vi "Autonomous Independent.vi"() -> ()   [LabVIEW 2016]
doc: "This VI is called when autonomous begins, and will automatically be terminated when autonomous ends. You can carry out timed or sensor driven robot movement independently without needing to return to the caller."
uses:
  <vilib>/Rock Robotics/WPI/Solenoid/WPI_SolenoidValue.ctl
  <vilib>/Rock Robotics/WPI/Utilities/WPI_GetSetVariantRefNum.vi
  <vilib>/Rock Robotics/Network Tables/NT Read String.vi
  <vilib>/Rock Robotics/WPI/RobotDrive/WPI_RobotDriveArcadeDrive_Standard(NoSaturation).vi
  <vilib>/Rock Robotics/Network Tables/NT Write Numeric Array.vi
  <vilib>/Rock Robotics/Network Tables/NT Read Number.vi
  <vilib>/Rock Robotics/WPI/Solenoid/WPI_SolenoidSetEnum.vi
  <vilib>/Rock Robotics/WPI/Solenoid/WPI_SolenoidGetEnum.vi
  <vilib>/addons/control/pid/pid.llb/PID (DBL).vi
  <vilib>/Rock Robotics/Network Tables/NT Write Number.vi
  <vilib>/addons/control/pid/NI_PID_pid.lvlib
panel:
  out "Boolean 3":bool=TRUE
  out "Boolean 2":bool=TRUE
  out "Boolean":bool=TRUE
  # "Be sure to right-click and choose Data Operations>>Make Current Value default if you want to save the array values with the VI"
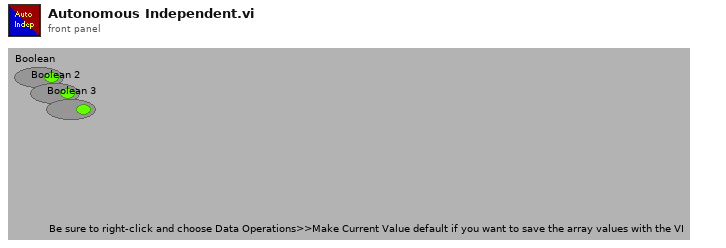
[diagram p1: front panel]
types:
  T1 = typedef "WPI_JoystickDevRef.ctl" = cluster{"Device":T2}
  T2 = typedef "WPI_JoystickDeviceEnum.ctl" = enum16{"USB 0", "USB 1", "USB 2", "USB 3", "USB 4", "USB 5"}
  T3 = typedef "WPI_SolenoidValue.ctl" = enum16{"Off", "On", "Forward", "Reverse"}
  T4 = cluster{"integral time (Ti, min)":dbl, "proportional gain (Kc)":dbl, "derivative time (Td, min)":dbl}
  T5 = cluster{"integral time (Ti, min)":dbl, "proportional gain (Kc)":dbl}
  T6 = typedef "WPI_RobotDriveDevRef.ctl" = cluster{"DevStatus":errorcluster, "Motors[]":T7[], "Square Inputs":bool, "Max Output":dbl}
  T7 = typedef "WPI_MotorControlDeviceRef.ctl" = cluster{"DeviceStatus":errorcluster, "Type":T8, "PWM":cluster{"PWM Channel":T9, "DeadBand":T10}, "CAN":cluster{"Device Number":u8, "SetOutput VI Ref":variant, "GetOutput VI Ref":variant, "Enable VI Ref":variant, "Disable VI Ref":variant, "Data":variant}, "Invert":bool}
  T8 = typedef "WPI_MotorControlType.ctl" = enum16{"PWM", "CAN"}
  T9 = typedef "FPGA_DIOPWMChannel.ctl" = enum8{"PWM 0", "PWM 1", "PWM 2", "PWM 3", "PWM 4", "PWM 5", "PWM 6", "PWM 7", "PWM 8", "PWM 9", "PWM MXP 0", "PWM MXP 1", "PWM MXP 2", "PWM MXP 3", "PWM MXP 4", "PWM MXP 5", "PWM MXP 6", "PWM MXP 7", "PWM MXP 8", "PWM MXP 9", "Invalid"}
  T10 = typedef "WPI_PWMDeadband.ctl" = cluster{"Name":string, "maxPositivePwm":i32, "minPositivePwm":i32, "centerPwm":i32, "maxNegativePwm":i32, "minNegativePwm":i32, "angularRange":u16}
  T11 = typedef "WPI_SolenoidDevRef.ctl" = cluster{"DevStatus":errorcluster, "Pneumatics Control Module":u8, "Forward Solenoid Channel":T12, "Reverse Solenoid Channel":T12}
  T12 = typedef "WPI_SolenoidChannel.ctl" = enum8{"Solenoid 0", "Solenoid 1", "Solenoid 2", "Solenoid 3", "Solenoid 4", "Solenoid 5", "Solenoid 6", "Solenoid 7", "Invalid"}
  T13 = typedef "WPI_GyroDevRef.ctl" = cluster{"DevStatus":errorcluster, "Analog Channel":T14, "Offset":dbl, "Gain (VoltsPerDegree/Second)":dbl, "Gyro Type":enum16{"Analog", "XRS450"}, "Handle":i32, "SPI Bus":T15, "Device Found":bool, "Sample Rate":dbl, "Calibrate On Open":bool}
  T14 = typedef "FPGA_AIChannel.ctl" = enum8{"AI 0", "AI 1", "AI 2", "AI 3", "AI MXP 0", "AI MXP 1", "AI MXP 2", "AI MXP 3", "Invalid"}
  T15 = typedef "spi_bus.ctl" = enum16{"SPI On-Board, CS0", "SPI On-Board, CS1", "SPI On-Board, CS2", "SPI On-Board, CS3", "SPI MXP", "Invalid"}
  T16 = cluster{"Numeric":dbl, "Numeric":dbl, "Numeric":dbl}
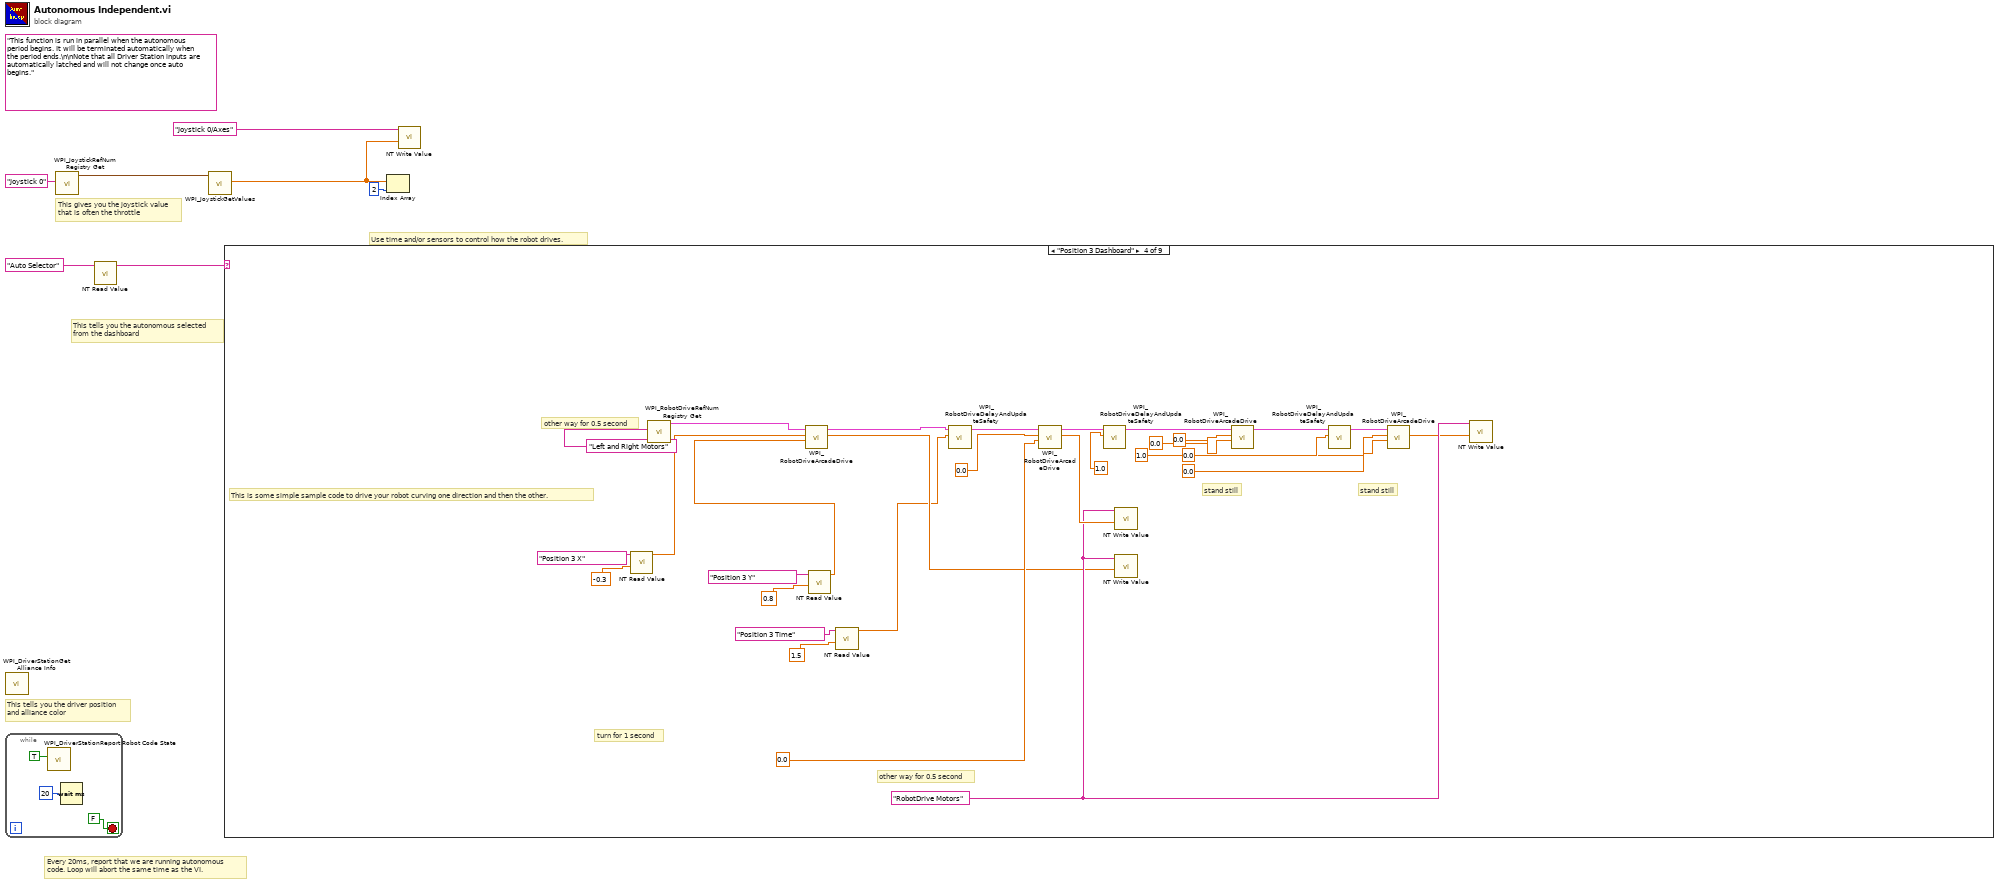
[diagram p0: block diagram]
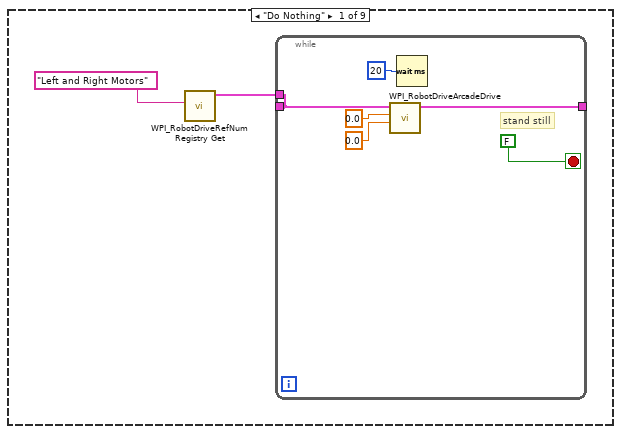
[diagram p2: hidden frame]
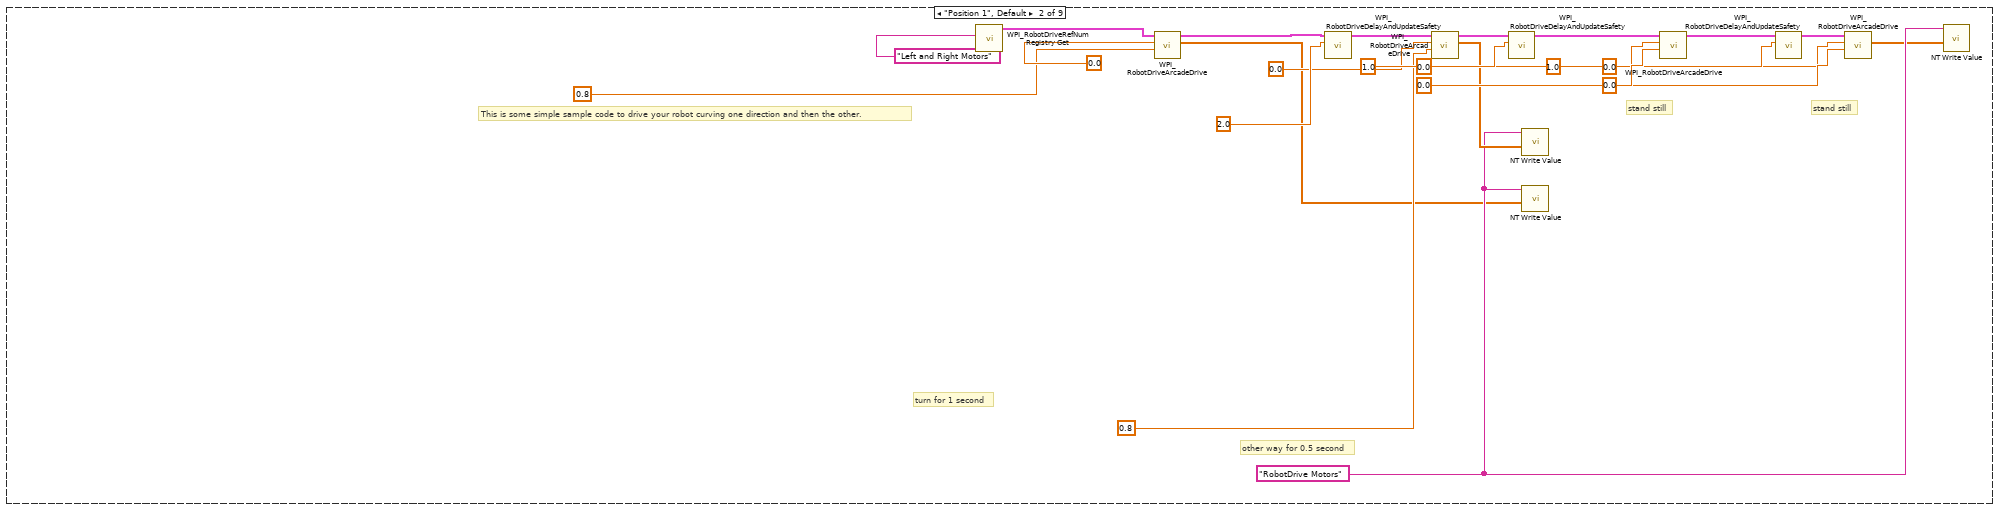
[diagram p3: hidden frame]
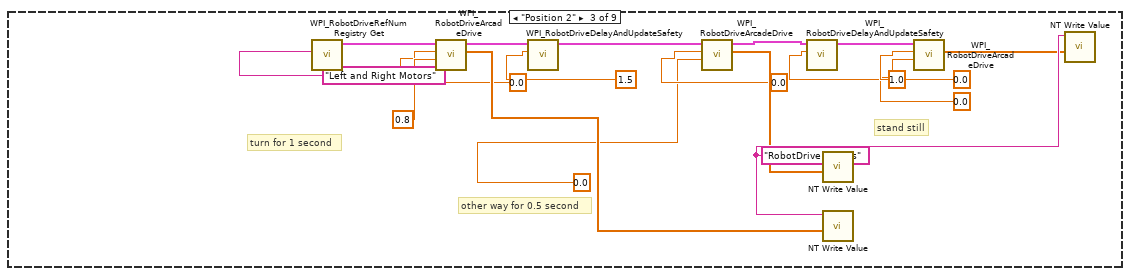
[diagram p4: hidden frame]
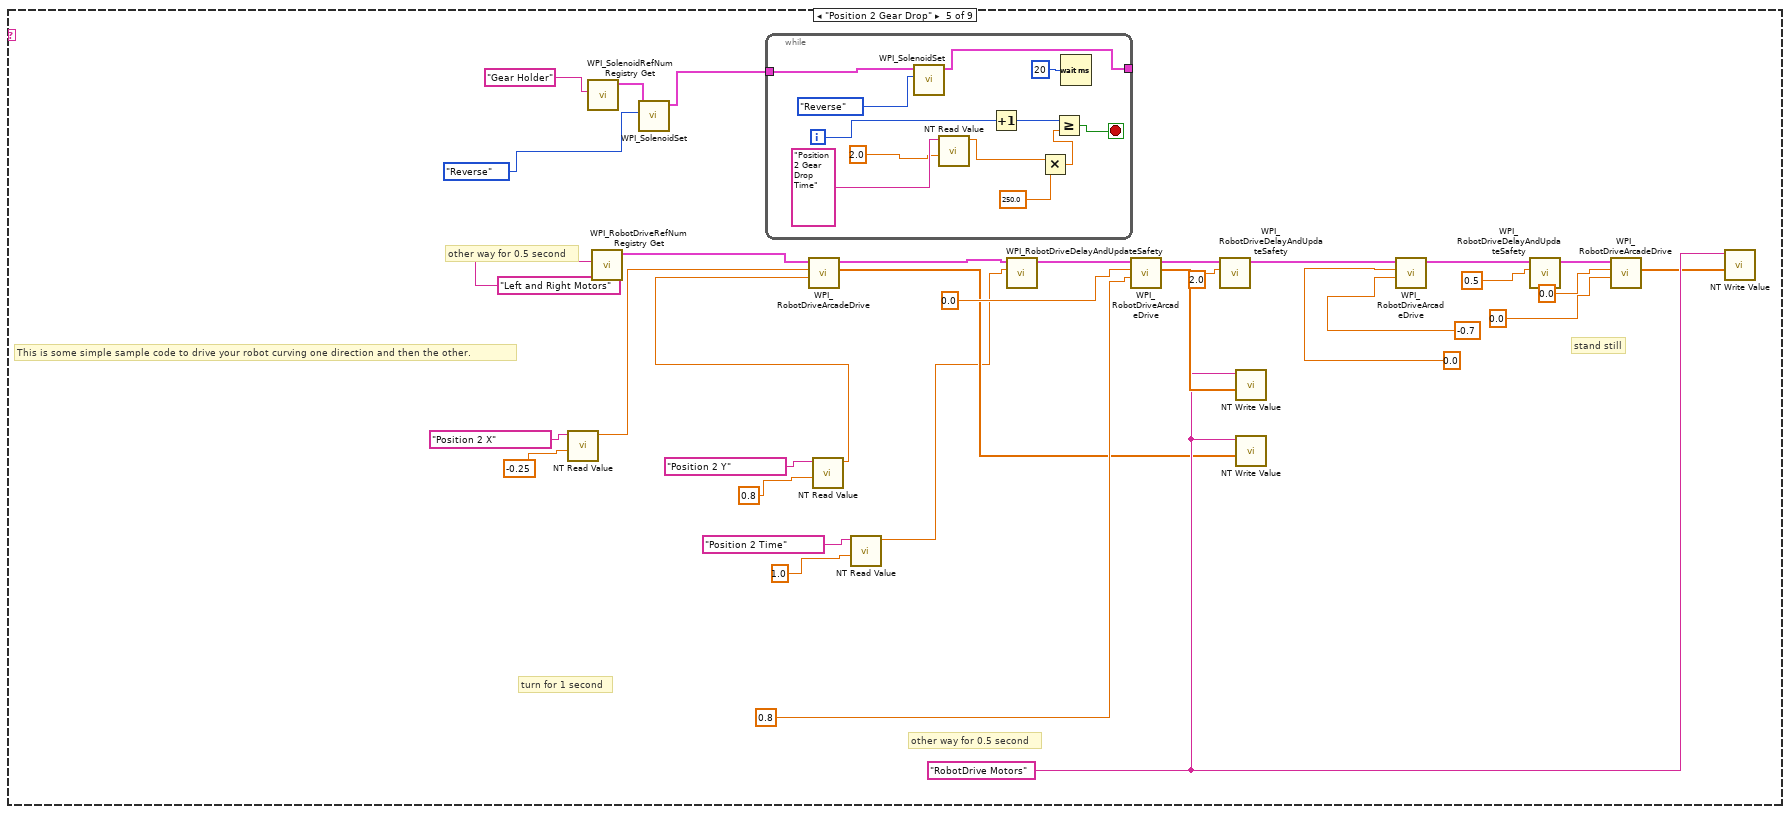
[diagram p5: hidden frame]
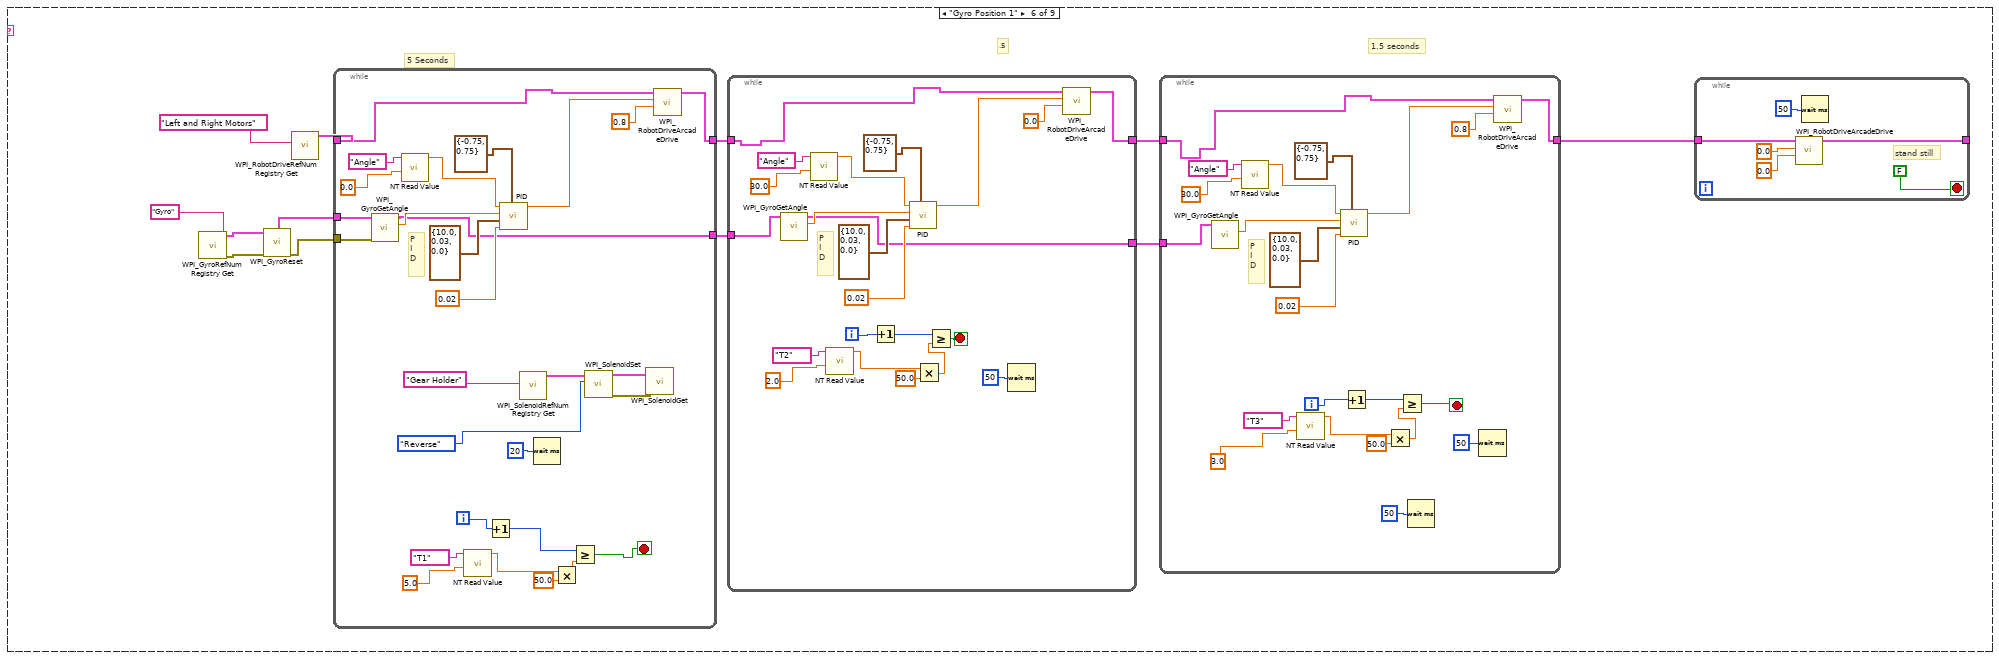
[diagram p6: hidden frame]
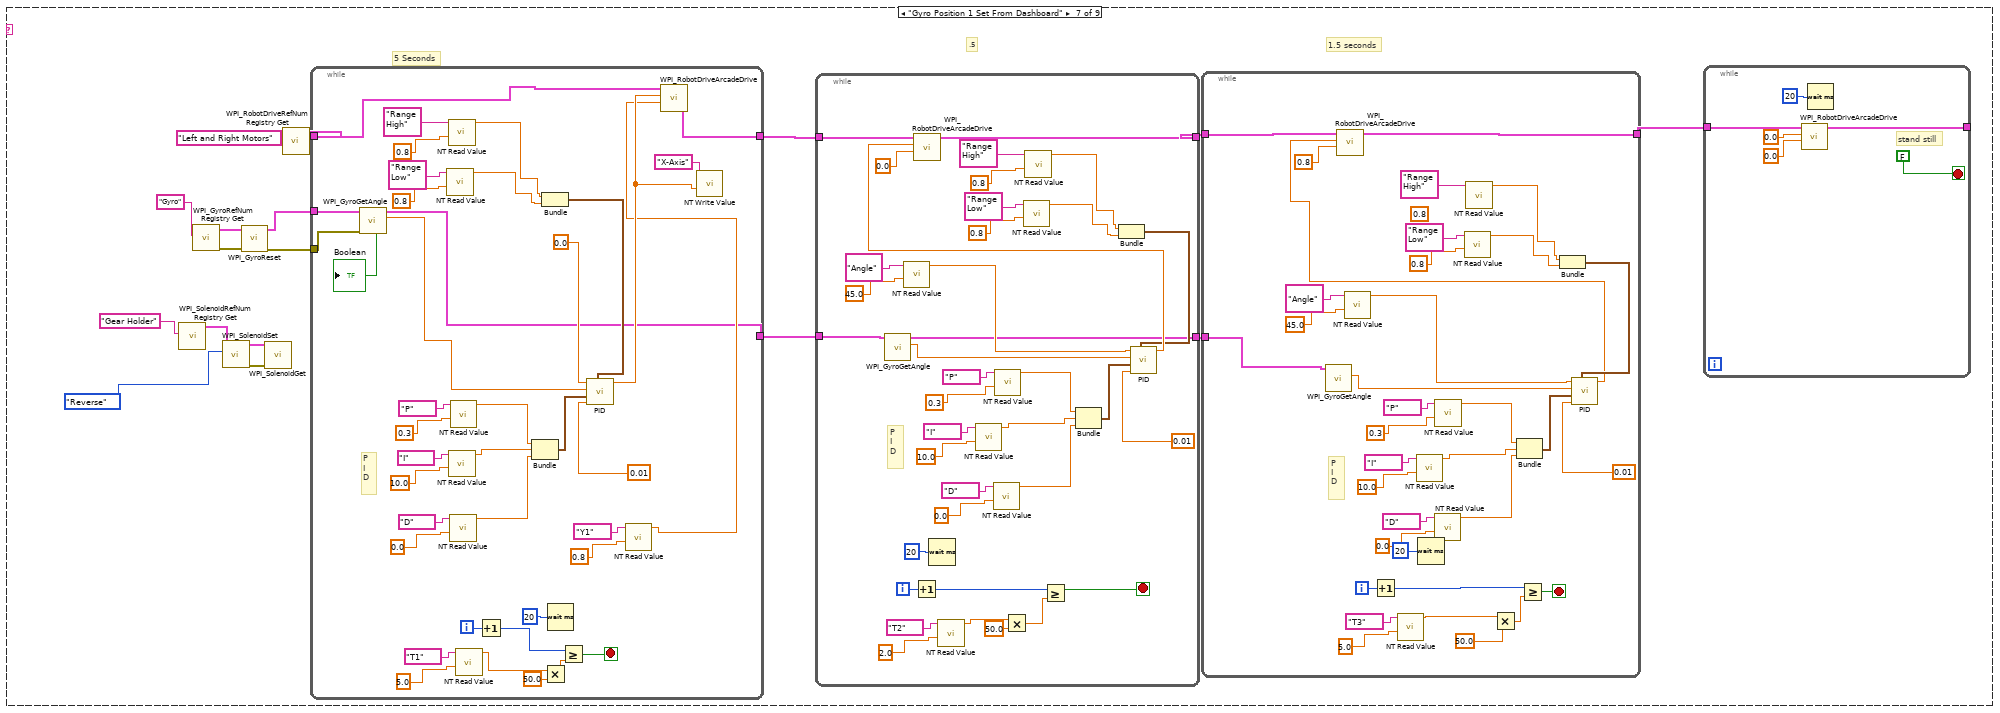
[diagram p7: hidden frame]
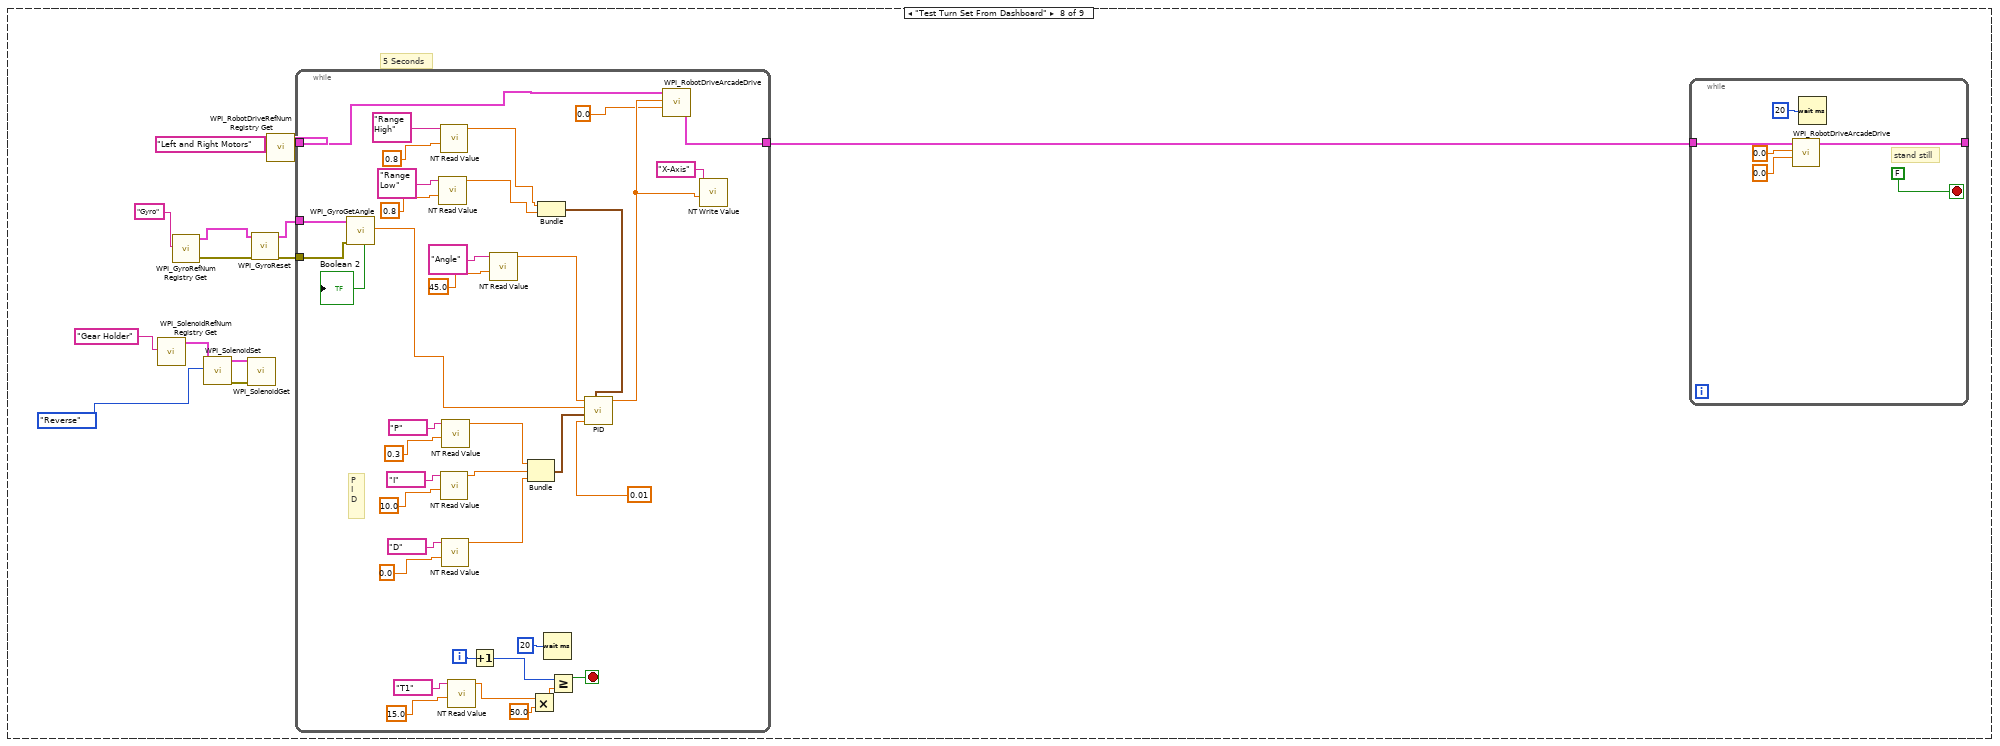
[diagram p8: hidden frame]
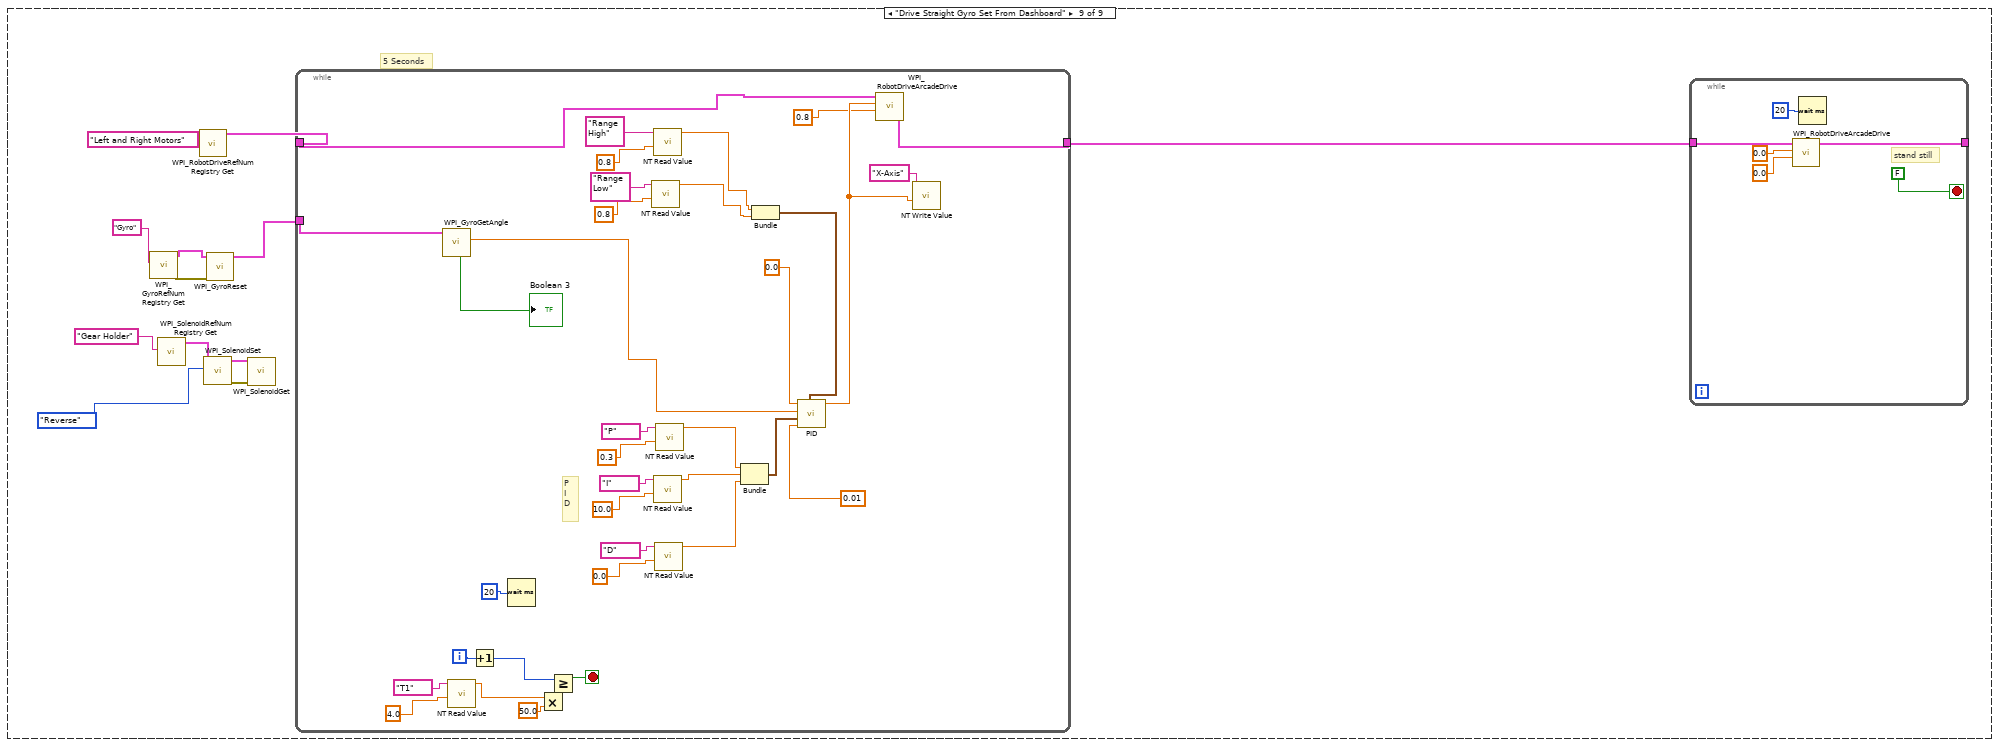
[diagram p9: hidden frame]
diagram:
  (unwired) "This function is run in parallel when the autonomous period begins. It will be terminated automatically when the period ends.\n\nNote that all Driver Station inputs are automatically latched and will not change once auto begins."
  # "This tells you the autonomous selected\nfrom the dashboard"
  # "Every 20ms, report that we are running autonomous\ncode. Loop will abort the same time as the VI."
  # "This gives you the joystick value\nthat is often the throttle"
  # "Use time and/or sensors to control how the robot drives."
  # "This tells you the driver position\nand alliance color"
  n1 = call <vilib>:"WPI_DriverStationGet Alliance Info.vi"() -> ()  [unwired: 12 out]
  n2 = while {
    stop <- FALSE stop-if-true
    n3 = call <vilib>:"WPI_DriverStationReport Robot Code State.vi"("Autonomous"=TRUE) -> ()  [unwired: 10 in, 1 out]
    n4 = Wait (ms)(milliseconds to wait=u32 20) -> ()  [unwired: 1 out]
  }
  n5 = call <vilib>:"WPI_JoystickRefNum Registry Get.vi"("refnum name"="Joystick 0") -> ("JoystickDevRef"=w6:T1)  [unwired: 1 in, 9 out]
  n6 = call-poly <vilib>:"NT Read Value.vi"("Name"="Auto Selector") -> ("String"=w3:string)  [unwired: 9 in, 1 out]
  n7 = call <vilib>:"WPI_JoystickGetValues.vi"("JoystickDevRef"=w6) -> ("Axes"=w2:dbl[])  [unwired: 6 in, 4 out]
  n8 = case shown="\"Position 3 Dashboard\"" w3 {
    frame "Do Nothing" {
      n9 = call <vilib>:"WPI_RobotDriveRefNum Registry Get.vi"("refnum name"="Left and Right Motors") -> ("RobotDriveDevRef"=w11:T6)  [unwired: 1 in, 9 out]
      n10 = while {
        tunnel: [w13] -> _
        tunnel: [w14] -> _
        tunnel: w11 -> [w13]
        stop <- FALSE stop-if-true
        # "stand still"
        n11 = call-poly <vilib>:"WPI_RobotDriveArcadeDrive.vi"("Y axis value"=0.0 ("X axis value"), "X axis value"=0.0, "RobotDriveDevRef"=w13) -> ("RobotDriveDevRef"=w14:T6)  [unwired: 1 in, 7 out]
        n12 = Wait (ms)(milliseconds to wait=20) -> ()  [unwired: 1 out]
      }
    }
    frame "Position 1", Default {
      w26 = "RobotDrive Motors" ("Name")
      # "stand still"
      # "stand still"
      # "other way for 0.5 second"
      # "turn for 1 second"
      # "This is some simple sample code to drive your robot curving one direction and then the other."
      n13 = call <vilib>:"WPI_RobotDriveRefNum Registry Get.vi"("refnum name"="Left and Right Motors") -> ("RobotDriveDevRef"=w41:T6)  [unwired: 1 in, 9 out]
      n14 = call-poly <vilib>:"WPI_RobotDriveArcadeDrive.vi"("Y axis value"=0.8 ("X axis value"), "X axis value"=0.0, "RobotDriveDevRef"=w41) -> ("Motor Values"=w25:dbl[], "RobotDriveDevRef"=w34:T6)  [unwired: 1 in, 6 out]
      n15 = call <vilib>:"WPI_RobotDriveDelayAndUpdateSafety.vi"("Delay (s)"=2.0, "RobotDriveDevRef"=w34) -> ("RobotDriveDevRef 2"=w35:T6)  [unwired: 8 in, 1 out]
      n16 = call-poly <vilib>:"WPI_RobotDriveArcadeDrive.vi"("Y axis value"=0.8 ("X axis value"), "X axis value"=0.0, "RobotDriveDevRef"=w35) -> ("Motor Values"=w27:dbl[], "RobotDriveDevRef"=w36:T6)  [unwired: 1 in, 6 out]
      n17 = call <vilib>:"WPI_RobotDriveDelayAndUpdateSafety.vi"("Delay (s)"=1.0, "RobotDriveDevRef"=w36) -> ("RobotDriveDevRef 2"=w37:T6)  [unwired: 8 in, 1 out]
      n18 = call-poly <vilib>:"NT Write Value.vi"("Numeric Array"=w27, "Name"=w26) -> ()  [unwired: 9 in, 1 out]
      n19 = call-poly <vilib>:"NT Write Value.vi"("Numeric Array"=w25, "Name"=w26) -> ()  [unwired: 9 in, 1 out]
      n20 = call-poly <vilib>:"WPI_RobotDriveArcadeDrive.vi"("Y axis value"=0.0 ("X axis value"), "X axis value"=0.0, "RobotDriveDevRef"=w37) -> ("RobotDriveDevRef"=w23:T6)  [unwired: 1 in, 7 out]
      n21 = call <vilib>:"WPI_RobotDriveDelayAndUpdateSafety.vi"("Delay (s)"=1.0, "RobotDriveDevRef"=w23) -> ("RobotDriveDevRef 2"=w21:T6)  [unwired: 8 in, 1 out]
      n22 = call-poly <vilib>:"WPI_RobotDriveArcadeDrive.vi"("Y axis value"=0.0 ("X axis value"), "X axis value"=0.0, "RobotDriveDevRef"=w21) -> ("Motor Values"=w20:dbl[])  [unwired: 1 in, 7 out]
      n23 = call-poly <vilib>:"NT Write Value.vi"("Numeric Array"=w20, "Name"=w26) -> ()  [unwired: 9 in, 1 out]
    }
    frame "Position 2" {
      w58 = "RobotDrive Motors" ("Name")
      # "stand still"
      # "other way for 0.5 second"
      # "turn for 1 second"
      n24 = call <vilib>:"WPI_RobotDriveRefNum Registry Get.vi"("refnum name"="Left and Right Motors") -> ("RobotDriveDevRef"=w42:T6)  [unwired: 1 in, 9 out]
      n25 = call-poly <vilib>:"WPI_RobotDriveArcadeDrive.vi"("Y axis value"=0.8 ("X axis value"), "X axis value"=0.0, "RobotDriveDevRef"=w42) -> ("Motor Values"=w59:dbl[], "RobotDriveDevRef"=w49:T6)  [unwired: 1 in, 6 out]
      n26 = call <vilib>:"WPI_RobotDriveDelayAndUpdateSafety.vi"("Delay (s)"=1.5, "RobotDriveDevRef"=w49) -> ("RobotDriveDevRef 2"=w48:T6)  [unwired: 8 in, 1 out]
      n27 = call-poly <vilib>:"WPI_RobotDriveArcadeDrive.vi"("Y axis value"=0.0 ("X axis value"), "X axis value"=0.0, "RobotDriveDevRef"=w48) -> ("Motor Values"=w57:dbl[], "RobotDriveDevRef"=w47:T6)  [unwired: 1 in, 6 out]
      n28 = call <vilib>:"WPI_RobotDriveDelayAndUpdateSafety.vi"("Delay (s)"=1.0, "RobotDriveDevRef"=w47) -> ("RobotDriveDevRef 2"=w46:T6)  [unwired: 8 in, 1 out]
      n29 = call-poly <vilib>:"NT Write Value.vi"("Numeric Array"=w57, "Name"=w58) -> ()  [unwired: 9 in, 1 out]
      n30 = call-poly <vilib>:"NT Write Value.vi"("Numeric Array"=w59, "Name"=w58) -> ()  [unwired: 9 in, 1 out]
      n31 = call-poly <vilib>:"WPI_RobotDriveArcadeDrive.vi"("Y axis value"=0.0 ("X axis value"), "X axis value"=0.0, "RobotDriveDevRef"=w46) -> ("Motor Values"=w56:dbl[])  [unwired: 1 in, 7 out]
      n32 = call-poly <vilib>:"NT Write Value.vi"("Numeric Array"=w56, "Name"=w58) -> ()  [unwired: 9 in, 1 out]
    }
    frame "Position 3 Dashboard" {
      w76 = "RobotDrive Motors" ("Name")
      # "stand still"
      # "stand still"
      # "other way for 0.5 second"
      # "turn for 1 second"
      # "This is some simple sample code to drive your robot curving one direction and then the other."
      # "other way for 0.5 second"
      n33 = call-poly <vilib>:"NT Read Value.vi"("Default Value"=-0.3, "Name"="Position 3 X" ("refnum name")) -> ("Numeric"=w66:dbl)  [unwired: 8 in, 1 out]
      n34 = call <vilib>:"WPI_RobotDriveRefNum Registry Get.vi"("refnum name"="Left and Right Motors") -> ("RobotDriveDevRef"=w88:T6)  [unwired: 1 in, 9 out]
      n35 = call-poly <vilib>:"NT Read Value.vi"("Default Value"=0.8, "Name"="Position 3 Y" ("refnum name")) -> ("Numeric"=w63:dbl)  [unwired: 8 in, 1 out]
      n36 = call-poly <vilib>:"WPI_RobotDriveArcadeDrive.vi"("Y axis value"=w63, "X axis value"=w66, "RobotDriveDevRef"=w88) -> ("Motor Values"=w75:dbl[], "RobotDriveDevRef"=w82:T6)  [unwired: 1 in, 6 out]
      n37 = call-poly <vilib>:"NT Read Value.vi"("Default Value"=1.5, "Name"="Position 3 Time" ("refnum name")) -> ("Numeric"=w60:dbl)  [unwired: 8 in, 1 out]
      n38 = call <vilib>:"WPI_RobotDriveDelayAndUpdateSafety.vi"("Delay (s)"=w60, "RobotDriveDevRef"=w82) -> ("RobotDriveDevRef 2"=w83:T6)  [unwired: 8 in, 1 out]
      n39 = call-poly <vilib>:"WPI_RobotDriveArcadeDrive.vi"("Y axis value"=0.0 ("X axis value"), "X axis value"=0.0, "RobotDriveDevRef"=w83) -> ("Motor Values"=w77:dbl[], "RobotDriveDevRef"=w84:T6)  [unwired: 1 in, 6 out]
      n40 = call <vilib>:"WPI_RobotDriveDelayAndUpdateSafety.vi"("Delay (s)"=1.0, "RobotDriveDevRef"=w84) -> ("RobotDriveDevRef 2"=w85:T6)  [unwired: 8 in, 1 out]
      n41 = call-poly <vilib>:"NT Write Value.vi"("Numeric Array"=w77, "Name"=w76) -> ()  [unwired: 9 in, 1 out]
      n42 = call-poly <vilib>:"NT Write Value.vi"("Numeric Array"=w75, "Name"=w76) -> ()  [unwired: 9 in, 1 out]
      n43 = call-poly <vilib>:"WPI_RobotDriveArcadeDrive.vi"("Y axis value"=0.0 ("X axis value"), "X axis value"=0.0, "RobotDriveDevRef"=w85) -> ("RobotDriveDevRef"=w73:T6)  [unwired: 1 in, 7 out]
      n44 = call <vilib>:"WPI_RobotDriveDelayAndUpdateSafety.vi"("Delay (s)"=1.0, "RobotDriveDevRef"=w73) -> ("RobotDriveDevRef 2"=w71:T6)  [unwired: 8 in, 1 out]
      n45 = call-poly <vilib>:"WPI_RobotDriveArcadeDrive.vi"("Y axis value"=0.0 ("X axis value"), "X axis value"=0.0, "RobotDriveDevRef"=w71) -> ("Motor Values"=w70:dbl[])  [unwired: 1 in, 7 out]
      n46 = call-poly <vilib>:"NT Write Value.vi"("Numeric Array"=w70, "Name"=w76) -> ()  [unwired: 9 in, 1 out]
    }
    frame "Position 2 Gear Drop" {
      w109 = "RobotDrive Motors" ("Name")
      # "stand still"
      # "other way for 0.5 second"
      # "turn for 1 second"
      # "This is some simple sample code to drive your robot curving one direction and then the other."
      # "other way for 0.5 second"
      n47 = call-poly <vilib>:"NT Read Value.vi"("Default Value"=-0.25, "Name"="Position 2 X" ("refnum name")) -> ("Numeric"=w99:dbl)  [unwired: 8 in, 1 out]
      n48 = call <vilib>:"WPI_SolenoidRefNum Registry Get.vi"("refnum name"="Gear Holder") -> ("SolenoidDevRef"=w91:T11)  [unwired: 9 in, 1 out]
      n49 = call <vilib>:"WPI_RobotDriveRefNum Registry Get.vi"("refnum name"="Left and Right Motors") -> ("RobotDriveDevRef"=w121:T6)  [unwired: 1 in, 9 out]
      n50 = call-poly <vilib>:"WPI_SolenoidSet.vi"("Value"=WPI_SolenoidValue."Reverse", "SolenoidDevRef"=w91) -> ("SolenoidDevRef"=w89:T11)  [unwired: 8 in, 1 out]
      n51 = while {
        tunnel: w89 -> [w125]
        tunnel: [w123] -> _
        i -> [w127]
        stop <- w122 stop-if-true
        n52 = call-poly <vilib>:"WPI_SolenoidSet.vi"("Value"=WPI_SolenoidValue."Reverse", "SolenoidDevRef"=w125) -> ("SolenoidDevRef"=w123:T11)  [unwired: 8 in, 1 out]
        n53 = call-poly <vilib>:"NT Read Value.vi"("Default Value"=2.0, "Name"="Position 2 Gear Drop Time" ("refnum name")) -> ("Numeric"=w129:dbl)  [unwired: 8 in, 1 out]
        n54 = Increment(x=w127) -> (x+1=w128:i32)
        n55 = Multiply(x=w129, y=250.0) -> (x*y=w133:dbl)
        n56 = Greater Or Equal?(x=w128, y=w133) -> (x >= y?=w122:bool)
        n57 = Wait (ms)(milliseconds to wait=20) -> ()  [unwired: 1 out]
      }
      n58 = call-poly <vilib>:"NT Read Value.vi"("Default Value"=0.8, "Name"="Position 2 Y" ("refnum name")) -> ("Numeric"=w96:dbl)  [unwired: 8 in, 1 out]
      n59 = call-poly <vilib>:"WPI_RobotDriveArcadeDrive.vi"("Y axis value"=w96, "X axis value"=w99, "RobotDriveDevRef"=w121) -> ("Motor Values"=w108:dbl[], "RobotDriveDevRef"=w115:T6)  [unwired: 1 in, 6 out]
      n60 = call-poly <vilib>:"NT Read Value.vi"("Default Value"=1.0, "Name"="Position 2 Time" ("refnum name")) -> ("Numeric"=w93:dbl)  [unwired: 8 in, 1 out]
      n61 = call <vilib>:"WPI_RobotDriveDelayAndUpdateSafety.vi"("Delay (s)"=w93, "RobotDriveDevRef"=w115) -> ("RobotDriveDevRef 2"=w116:T6)  [unwired: 8 in, 1 out]
      n62 = call-poly <vilib>:"WPI_RobotDriveArcadeDrive.vi"("Y axis value"=0.8 ("X axis value"), "X axis value"=0.0, "RobotDriveDevRef"=w116) -> ("Motor Values"=w110:dbl[], "RobotDriveDevRef"=w117:T6)  [unwired: 1 in, 6 out]
      n63 = call <vilib>:"WPI_RobotDriveDelayAndUpdateSafety.vi"("Delay (s)"=2.0, "RobotDriveDevRef"=w117) -> ("RobotDriveDevRef 2"=w118:T6)  [unwired: 8 in, 1 out]
      n64 = call-poly <vilib>:"NT Write Value.vi"("Numeric Array"=w110, "Name"=w109) -> ()  [unwired: 9 in, 1 out]
      n65 = call-poly <vilib>:"NT Write Value.vi"("Numeric Array"=w108, "Name"=w109) -> ()  [unwired: 9 in, 1 out]
      n66 = call-poly <vilib>:"WPI_RobotDriveArcadeDrive.vi"("Y axis value"=-0.7 ("X axis value"), "X axis value"=0.0, "RobotDriveDevRef"=w118) -> ("RobotDriveDevRef"=w106:T6)  [unwired: 1 in, 7 out]
      n67 = call <vilib>:"WPI_RobotDriveDelayAndUpdateSafety.vi"("Delay (s)"=0.5, "RobotDriveDevRef"=w106) -> ("RobotDriveDevRef 2"=w104:T6)  [unwired: 8 in, 1 out]
      n68 = call-poly <vilib>:"WPI_RobotDriveArcadeDrive.vi"("Y axis value"=0.0 ("X axis value"), "X axis value"=0.0, "RobotDriveDevRef"=w104) -> ("Motor Values"=w103:dbl[])  [unwired: 1 in, 7 out]
      n69 = call-poly <vilib>:"NT Write Value.vi"("Numeric Array"=w103, "Name"=w109) -> ()  [unwired: 9 in, 1 out]
    }
    frame "Gyro Position 1" {
      # "1.5 seconds"
      # ".5"
      # "5 Seconds"
      n70 = call <vilib>:"WPI_GyroRefNum Registry Get.vi"("refnum name"="Gyro") -> ("error out"=w138:errorcluster, "GyroDevRef"=w139:T13)  [unwired: 9 in]
      n71 = call <vilib>:"WPI_GyroReset.vi"("error in"=w138, "GyroDevRef"=w139) -> ("error out"=w136:errorcluster, "GyroDevRef"=w137:T13)  [unwired: 8 in]
      n72 = call <vilib>:"WPI_RobotDriveRefNum Registry Get.vi"("refnum name"="Left and Right Motors") -> ("RobotDriveDevRef"=w142:T6)  [unwired: 1 in, 9 out]
      n73 = while {
        tunnel: w142 -> [w171]
        tunnel: [w170] -> w141
        tunnel: w137 -> [w164]
        tunnel: w136 -> [w147]
        tunnel: [w146] -> w135
        i -> [w148]
        stop <- w149 stop-if-true
        # "P\nI\nD"
        n74 = call <vilib>:"WPI_GyroGetAngle.vi"("error in"=w147, "GyroDevRef"=w164) -> ("Angle"=w163:dbl, "GyroDevRef"=w146:T13)  [unwired: 5 in, 3 out]
        n75 = call-poly <vilib>:"NT Read Value.vi"("Default Value"=0.0, "Name"="Angle" ("refnum name")) -> ("Numeric"=w158:dbl)  [unwired: 8 in, 1 out]
        n76 = call-poly <vilib>:"NT Read Value.vi"("Default Value"=5.0, "Name"="T1" ("refnum name")) -> ("Numeric"=w150:dbl)  [unwired: 8 in, 1 out]
        n77 = Increment(x=w148) -> (x+1=w155:i32)
        n78 = call-poly <vilib>:"PID.vi"("output range"=T5 {"integral time (Ti, min)"=-0.75, "proportional gain (Kc)"=0.75} ("PID gains"), "dt (s)"=0.02 ("proportional gain (Kc)"), "PID gains"=T4 {"integral time (Ti, min)"=10.0, "proportional gain (Kc)"=0.03, "derivative time (Td, min)"=0.0}, "process variable"=w163, "setpoint"=w158) -> ("output"=w159:dbl)  [unwired: 5 in, 1 out]
        n79 = call <vilib>:"WPI_SolenoidRefNum Registry Get.vi"("refnum name"="Gear Holder") -> ("SolenoidDevRef"=w169:T11)  [unwired: 9 in, 1 out]
        n80 = Wait (ms)(milliseconds to wait=20) -> ()  [unwired: 1 out]
        n81 = Multiply(x=w150, y=50.0) -> (x*y=w151:dbl)
        n82 = Greater Or Equal?(x=w155, y=w151) -> (x >= y?=w149:bool)
        n83 = call-poly <vilib>:"WPI_SolenoidSet.vi"("Value"=WPI_SolenoidValue."Reverse", "SolenoidDevRef"=w169) -> ("error out"=w167:errorcluster, "SolenoidDevRef"=w168:T11)  [unwired: 8 in]
        n84 = call-poly <vilib>:"WPI_SolenoidGet.vi"("error in (no error)"=w167, "SolenoidDevRef"=w168) -> ()  [unwired: 7 in, 3 out]
        n85 = call-poly <vilib>:"WPI_RobotDriveArcadeDrive.vi"("Y axis value"=0.8 ("X axis value"), "X axis value"=w159, "RobotDriveDevRef"=w171) -> ("RobotDriveDevRef"=w170:T6)  [unwired: 1 in, 7 out]
      }
      n86 = while {
        tunnel: w141 -> [w204]
        tunnel: [w203] -> w144
        tunnel: w135 -> [w205]
        tunnel: [w202] -> w134
        i -> [w223]
        stop <- w221 stop-if-true
        # "P\nI\nD"
        n87 = call <vilib>:"WPI_GyroGetAngle.vi"("GyroDevRef"=w205) -> ("Angle"=w207:dbl, "GyroDevRef"=w202:T13)  [unwired: 6 in, 3 out]
        n88 = call-poly <vilib>:"NT Read Value.vi"("Default Value"=30.0, "Name"="Angle" ("refnum name")) -> ("Numeric"=w212:dbl)  [unwired: 8 in, 1 out]
        n89 = call-poly <vilib>:"NT Read Value.vi"("Default Value"=2.0, "Name"="T2" ("refnum name")) -> ("Numeric"=w219:dbl)  [unwired: 8 in, 1 out]
        n90 = Increment(x=w223) -> (x+1=w222:i32)
        n91 = call-poly <vilib>:"PID.vi"("output range"=T5 {"integral time (Ti, min)"=-0.75, "proportional gain (Kc)"=0.75} ("PID gains"), "dt (s)"=0.02 ("proportional gain (Kc)"), "PID gains"=T4 {"integral time (Ti, min)"=10.0, "proportional gain (Kc)"=0.03, "derivative time (Td, min)"=0.0}, "process variable"=w207, "setpoint"=w212) -> ("output"=w211:dbl)  [unwired: 5 in, 1 out]
        n92 = Multiply(x=w219, y=50.0) -> (x*y=w215:dbl)
        n93 = Greater Or Equal?(x=w222, y=w215) -> (x >= y?=w221:bool)
        n94 = Wait (ms)(milliseconds to wait=50) -> ()  [unwired: 1 out]
        n95 = call-poly <vilib>:"WPI_RobotDriveArcadeDrive.vi"("Y axis value"=0.0 ("X axis value"), "X axis value"=w211, "RobotDriveDevRef"=w204) -> ("RobotDriveDevRef"=w203:T6)  [unwired: 1 in, 7 out]
      }
      n96 = while {
        tunnel: [w183] -> w143
        tunnel: w144 -> [w184]
        tunnel: w134 -> [w180]
        i -> [w182]
        stop <- w181 stop-if-true
        # "P\nI\nD"
        n97 = call <vilib>:"WPI_GyroGetAngle.vi"("GyroDevRef"=w180) -> ("Angle"=w199:dbl)  [unwired: 6 in, 4 out]
        n98 = call-poly <vilib>:"NT Read Value.vi"("Default Value"=30.0, "Name"="Angle" ("refnum name")) -> ("Numeric"=w194:dbl)  [unwired: 8 in, 1 out]
        n99 = call-poly <vilib>:"NT Read Value.vi"("Default Value"=3.0, "Name"="T3" ("refnum name")) -> ("Numeric"=w187:dbl)  [unwired: 8 in, 1 out]
        n100 = call-poly <vilib>:"PID.vi"("output range"=T5 {"integral time (Ti, min)"=-0.75, "proportional gain (Kc)"=0.75} ("PID gains"), "dt (s)"=0.02 ("proportional gain (Kc)"), "PID gains"=T4 {"integral time (Ti, min)"=10.0, "proportional gain (Kc)"=0.03, "derivative time (Td, min)"=0.0}, "process variable"=w199, "setpoint"=w194) -> ("output"=w195:dbl)  [unwired: 5 in, 1 out]
        n101 = Increment(x=w182) -> (x+1=w185:i32)
        n102 = Multiply(x=w187, y=50.0) -> (x*y=w191:dbl)
        n103 = Greater Or Equal?(x=w185, y=w191) -> (x >= y?=w181:bool)
        n104 = Wait (ms)(milliseconds to wait=50) -> ()  [unwired: 1 out]
        n105 = Wait (ms)(milliseconds to wait=50) -> ()  [unwired: 1 out]
        n106 = call-poly <vilib>:"WPI_RobotDriveArcadeDrive.vi"("Y axis value"=0.8 ("X axis value"), "X axis value"=w195, "RobotDriveDevRef"=w184) -> ("RobotDriveDevRef"=w183:T6)  [unwired: 1 in, 7 out]
      }
      n107 = while {
        tunnel: w143 -> [w175]
        tunnel: [w174] -> _
        stop <- FALSE stop-if-true
        # "stand still"
        n108 = call-poly <vilib>:"WPI_RobotDriveArcadeDrive.vi"("Y axis value"=0.0 ("X axis value"), "X axis value"=0.0, "RobotDriveDevRef"=w175) -> ("RobotDriveDevRef"=w174:T6)  [unwired: 1 in, 7 out]
        n109 = Wait (ms)(milliseconds to wait=50) -> ()  [unwired: 1 out]
      }
    }
    frame "Gyro Position 1 Set From Dashboard" {
      # "1.5 seconds"
      # ".5"
      # "5 Seconds"
      n110 = call <vilib>:"WPI_SolenoidRefNum Registry Get.vi"("refnum name"="Gear Holder") -> ("SolenoidDevRef"=w231:T11)  [unwired: 9 in, 1 out]
      n111 = call <vilib>:"WPI_GyroRefNum Registry Get.vi"("refnum name"="Gyro") -> ("error out"=w225:errorcluster, "GyroDevRef"=w226:T13)  [unwired: 9 in]
      n112 = call-poly <vilib>:"WPI_SolenoidSet.vi"("Value"=WPI_SolenoidValue."Reverse", "SolenoidDevRef"=w231) -> ("error out"=w233:errorcluster, "SolenoidDevRef"=w232:T11)  [unwired: 8 in]
      n113 = call <vilib>:"WPI_GyroReset.vi"("error in"=w225, "GyroDevRef"=w226) -> ("error out"=w224:errorcluster, "GyroDevRef"=w227:T13)  [unwired: 8 in]
      n114 = call-poly <vilib>:"WPI_SolenoidGet.vi"("error in (no error)"=w233, "SolenoidDevRef"=w232) -> ()  [unwired: 7 in, 3 out]
      n115 = call <vilib>:"WPI_RobotDriveRefNum Registry Get.vi"("refnum name"="Left and Right Motors") -> ("RobotDriveDevRef"=w237:T6)  [unwired: 1 in, 9 out]
      n116 = while {
        tunnel: w237 -> [w276]
        tunnel: [w275] -> w236
        tunnel: w227 -> [w241]
        tunnel: [w246] -> w229
        tunnel: w224 -> [w242]
        i -> [w279]
        stop <- w277 stop-if-true
        # "P\nI\nD"
        n117 = call <vilib>:"WPI_GyroGetAngle.vi"("error in"=w242, "GyroDevRef"=w241) -> ("Angle"=w253:dbl, "GyroDevRef"=w246:T13, "Calibrated?"=→"Boolean":bool)  [unwired: 5 in, 2 out]
        n118 = call-poly <vilib>:"NT Read Value.vi"("Default Value"=0.8, "Name"="Range Low" ("refnum name")) -> ("Numeric"=w268:dbl)  [unwired: 8 in, 1 out]
        n119 = call-poly <vilib>:"NT Read Value.vi"("Default Value"=0.8, "Name"="Range High" ("refnum name")) -> ("Numeric"=w269:dbl)  [unwired: 8 in, 1 out]
        n120 = call-poly <vilib>:"NT Read Value.vi"("Default Value"=10.0, "Name"="I" ("refnum name")) -> ("Numeric"=w260:dbl)  [unwired: 8 in, 1 out]
        n121 = call-poly <vilib>:"NT Read Value.vi"("Default Value"=0.0, "Name"="D" ("refnum name")) -> ("Numeric"=w259:dbl)  [unwired: 8 in, 1 out]
        n122 = call-poly <vilib>:"NT Read Value.vi"("Default Value"=0.3, "Name"="P" ("refnum name")) -> ("Numeric"=w258:dbl)  [unwired: 8 in, 1 out]
        n123 = call-poly <vilib>:"NT Read Value.vi"("Default Value"=5.0, "Name"="T1" ("refnum name")) -> ("Numeric"=w243:dbl)  [unwired: 8 in, 1 out]
        n124 = Increment(x=w279) -> (x+1=w280:i32)
        n125 = Bundle("Numeric"=w258, "Numeric"=w260, "Numeric"=w259) -> (w257:T16)  [unwired: 1 in]
        n126 = Bundle("Numeric"=w269, "Numeric"=w268) -> (w267:cluster{"Numeric":dbl, "Numeric":dbl})  [unwired: 1 in]
        n127 = Multiply(x=w243, y=50.0) -> (x*y=w244:dbl)
        n128 = Wait (ms)(milliseconds to wait=20) -> ()  [unwired: 1 out]
        n129 = Greater Or Equal?(x=w280, y=w244) -> (x >= y?=w277:bool)
        n130 = call-poly <vilib>:"PID.vi"("output range"=w267, "dt (s)"=0.01 ("proportional gain (Kc)"), "PID gains"=w257, "process variable"=w253, "setpoint"=0.0) -> ("output"=w254:dbl)  [unwired: 5 in, 1 out]
        n131 = call-poly <vilib>:"NT Read Value.vi"("Default Value"=0.8, "Name"="Y1" ("refnum name")) -> ("Numeric"=w248:dbl)  [unwired: 8 in, 1 out]
        n132 = call-poly <vilib>:"WPI_RobotDriveArcadeDrive.vi"("Y axis value"=w248, "X axis value"=w254, "RobotDriveDevRef"=w276) -> ("RobotDriveDevRef"=w275:T6)  [unwired: 1 in, 7 out]
        n133 = call-poly <vilib>:"NT Write Value.vi"("Numeric"=w254, "Name"="X-Axis" ("refnum name")) -> ()  [unwired: 9 in, 1 out]
      }
      n134 = while {
        tunnel: w236 -> [w354]
        tunnel: [w352] -> w239
        tunnel: w229 -> [w327]
        tunnel: [w325] -> w228
        i -> [w358]
        stop <- w356 stop-if-true
        # "P\nI\nD"
        n135 = call <vilib>:"WPI_GyroGetAngle.vi"("GyroDevRef"=w327) -> ("Angle"=w326:dbl, "GyroDevRef"=w325:T13)  [unwired: 6 in, 3 out]
        n136 = call-poly <vilib>:"NT Read Value.vi"("Default Value"=45.0, "Name"="Angle" ("refnum name")) -> ("Numeric"=w328:dbl)  [unwired: 8 in, 1 out]
        n137 = Increment(x=w358) -> (x+1=w357:i32)
        n138 = Wait (ms)(milliseconds to wait=20) -> ()  [unwired: 1 out]
        n139 = call-poly <vilib>:"NT Read Value.vi"("Default Value"=2.0, "Name"="T2" ("refnum name")) -> ("Numeric"=w323:dbl)  [unwired: 8 in, 1 out]
        n140 = call-poly <vilib>:"NT Read Value.vi"("Default Value"=10.0, "Name"="I" ("refnum name")) -> ("Numeric"=w338:dbl)  [unwired: 8 in, 1 out]
        n141 = call-poly <vilib>:"NT Read Value.vi"("Default Value"=0.0, "Name"="D" ("refnum name")) -> ("Numeric"=w345:dbl)  [unwired: 8 in, 1 out]
        n142 = call-poly <vilib>:"NT Read Value.vi"("Default Value"=0.3, "Name"="P" ("refnum name")) -> ("Numeric"=w346:dbl)  [unwired: 8 in, 1 out]
        n143 = Multiply(x=w323, y=50.0) -> (x*y=w322:dbl)
        n144 = call-poly <vilib>:"NT Read Value.vi"("Default Value"=0.8, "Name"="Range Low" ("refnum name")) -> ("Numeric"=w335:dbl)  [unwired: 8 in, 1 out]
        n145 = call-poly <vilib>:"NT Read Value.vi"("Default Value"=0.8, "Name"="Range High" ("refnum name")) -> ("Numeric"=w334:dbl)  [unwired: 8 in, 1 out]
        n146 = Greater Or Equal?(x=w357, y=w322) -> (x >= y?=w356:bool)
        n147 = Bundle("Numeric"=w346, "Numeric"=w338, "Numeric"=w345) -> (w347:T16)  [unwired: 1 in]
        n148 = Bundle("Numeric"=w334, "Numeric"=w335) -> (w329:cluster{"Numeric":dbl, "Numeric":dbl})  [unwired: 1 in]
        n149 = call-poly <vilib>:"PID.vi"("output range"=w329, "dt (s)"=0.01 ("proportional gain (Kc)"), "PID gains"=w347, "process variable"=w326, "setpoint"=w328) -> ("output"=w336:dbl)  [unwired: 5 in, 1 out]
        n150 = call-poly <vilib>:"WPI_RobotDriveArcadeDrive.vi"("Y axis value"=0.0 ("X axis value"), "X axis value"=w336, "RobotDriveDevRef"=w354) -> ("RobotDriveDevRef"=w352:T6)  [unwired: 1 in, 7 out]
      }
      n151 = while {
        tunnel: [w321] -> w238
        tunnel: w239 -> [w319]
        tunnel: w228 -> [w290]
        i -> [w317]
        stop <- w316 stop-if-true
        (unwired) 0.8
        # "P\nI\nD"
        n152 = call <vilib>:"WPI_GyroGetAngle.vi"("GyroDevRef"=w290) -> ("Angle"=w312:dbl)  [unwired: 6 in, 4 out]
        n153 = call-poly <vilib>:"NT Read Value.vi"("Default Value"=45.0, "Name"="Angle" ("refnum name")) -> ("Numeric"=w311:dbl)  [unwired: 8 in, 1 out]
        n154 = Increment(x=w317) -> (x+1=w318:i32)
        n155 = call-poly <vilib>:"NT Read Value.vi"("Default Value"=5.0, "Name"="T3" ("refnum name")) -> ("Numeric"=w288:dbl)  [unwired: 8 in, 1 out]
        n156 = call-poly <vilib>:"NT Read Value.vi"("Default Value"=10.0, "Name"="I" ("refnum name")) -> ("Numeric"=w303:dbl)  [unwired: 8 in, 1 out]
        n157 = Wait (ms)(milliseconds to wait=20) -> ()  [unwired: 1 out]
        n158 = call-poly <vilib>:"NT Read Value.vi"("Default Value"=0.0, "Name"="D" ("refnum name")) -> ("Numeric"=w296:dbl)  [unwired: 8 in, 1 out]
        n159 = call-poly <vilib>:"NT Read Value.vi"("Default Value"=0.3, "Name"="P" ("refnum name")) -> ("Numeric"=w295:dbl)  [unwired: 8 in, 1 out]
        n160 = call-poly <vilib>:"NT Read Value.vi"("Default Value"=0.8, "Name"="Range Low" ("refnum name")) -> ("Numeric"=w305:dbl)  [unwired: 8 in, 1 out]
        n161 = call-poly <vilib>:"NT Read Value.vi"("Name"="Range High" ("refnum name")) -> ("Numeric"=w306:dbl)  [unwired: 9 in, 1 out]
        n162 = Multiply(x=w288, y=50.0) -> (x*y=w287:dbl)
        n163 = Bundle("Numeric"=w295, "Numeric"=w303, "Numeric"=w296) -> (w294:T16)  [unwired: 1 in]
        n164 = Greater Or Equal?(x=w318, y=w287) -> (x >= y?=w316:bool)
        n165 = Bundle("Numeric"=w306, "Numeric"=w305) -> (w310:cluster{"Numeric":dbl, "Numeric":dbl})  [unwired: 1 in]
        n166 = call-poly <vilib>:"PID.vi"("output range"=w310, "dt (s)"=0.01 ("proportional gain (Kc)"), "PID gains"=w294, "process variable"=w312, "setpoint"=w311) -> ("output"=w291:dbl)  [unwired: 5 in, 1 out]
        n167 = call-poly <vilib>:"WPI_RobotDriveArcadeDrive.vi"("Y axis value"=0.8 ("X axis value"), "X axis value"=w291, "RobotDriveDevRef"=w319) -> ("RobotDriveDevRef"=w321:T6)  [unwired: 1 in, 7 out]
      }
      n168 = while {
        tunnel: w238 -> [w282]
        tunnel: [w281] -> _
        stop <- FALSE stop-if-true
        # "stand still"
        n169 = call-poly <vilib>:"WPI_RobotDriveArcadeDrive.vi"("Y axis value"=0.0 ("X axis value"), "X axis value"=0.0, "RobotDriveDevRef"=w282) -> ("RobotDriveDevRef"=w281:T6)  [unwired: 1 in, 7 out]
        n170 = Wait (ms)(milliseconds to wait=20) -> ()  [unwired: 1 out]
      }
    }
    frame "Test Turn Set From Dashboard" {
      # "5 Seconds"
      n171 = call <vilib>:"WPI_SolenoidRefNum Registry Get.vi"("refnum name"="Gear Holder") -> ("SolenoidDevRef"=w365:T11)  [unwired: 9 in, 1 out]
      n172 = call <vilib>:"WPI_GyroRefNum Registry Get.vi"("refnum name"="Gyro") -> ("error out"=w359:errorcluster, "GyroDevRef"=w362:T13)  [unwired: 9 in]
      n173 = call-poly <vilib>:"WPI_SolenoidSet.vi"("Value"=WPI_SolenoidValue."Reverse", "SolenoidDevRef"=w365) -> ("error out"=w367:errorcluster, "SolenoidDevRef"=w366:T11)  [unwired: 8 in]
      n174 = call-poly <vilib>:"WPI_SolenoidGet.vi"("error in (no error)"=w367, "SolenoidDevRef"=w366) -> ()  [unwired: 7 in, 3 out]
      n175 = call <vilib>:"WPI_GyroReset.vi"("error in"=w359, "GyroDevRef"=w362) -> ("error out"=w360:errorcluster, "GyroDevRef"=w361:T13)  [unwired: 8 in]
      n176 = call <vilib>:"WPI_RobotDriveRefNum Registry Get.vi"("refnum name"="Left and Right Motors") -> ("RobotDriveDevRef"=w370:T6)  [unwired: 1 in, 9 out]
      n177 = while {
        tunnel: w370 -> [w406]
        tunnel: [w405] -> w363
        tunnel: w361 -> [w373]
        tunnel: w360 -> [w372]
        i -> [w409]
        stop <- w407 stop-if-true
        # "P\nI\nD"
        n178 = call <vilib>:"WPI_GyroGetAngle.vi"("error in"=w372, "GyroDevRef"=w373) -> ("Angle"=w383:dbl, "Calibrated?"=→"Boolean 2":bool)  [unwired: 5 in, 3 out]
        n179 = call-poly <vilib>:"NT Read Value.vi"("Default Value"=0.8, "Name"="Range Low" ("refnum name")) -> ("Numeric"=w398:dbl)  [unwired: 8 in, 1 out]
        n180 = call-poly <vilib>:"NT Read Value.vi"("Default Value"=0.8, "Name"="Range High" ("refnum name")) -> ("Numeric"=w399:dbl)  [unwired: 8 in, 1 out]
        n181 = call-poly <vilib>:"NT Read Value.vi"("Default Value"=10.0, "Name"="I" ("refnum name")) -> ("Numeric"=w390:dbl)  [unwired: 8 in, 1 out]
        n182 = call-poly <vilib>:"NT Read Value.vi"("Default Value"=0.0, "Name"="D" ("refnum name")) -> ("Numeric"=w389:dbl)  [unwired: 8 in, 1 out]
        n183 = call-poly <vilib>:"NT Read Value.vi"("Default Value"=0.3, "Name"="P" ("refnum name")) -> ("Numeric"=w388:dbl)  [unwired: 8 in, 1 out]
        n184 = call-poly <vilib>:"NT Read Value.vi"("Default Value"=15.0, "Name"="T1" ("refnum name")) -> ("Numeric"=w375:dbl)  [unwired: 8 in, 1 out]
        n185 = Increment(x=w409) -> (x+1=w410:i32)
        n186 = call-poly <vilib>:"NT Read Value.vi"("Default Value"=45.0, "Name"="Angle" ("refnum name")) -> ("Numeric"=w377:dbl)  [unwired: 8 in, 1 out]
        n187 = Bundle("Numeric"=w388, "Numeric"=w390, "Numeric"=w389) -> (w387:T16)  [unwired: 1 in]
        n188 = Multiply(x=w375, y=50.0) -> (x*y=w374:dbl)
        n189 = Bundle("Numeric"=w399, "Numeric"=w398) -> (w397:cluster{"Numeric":dbl, "Numeric":dbl})  [unwired: 1 in]
        n190 = Wait (ms)(milliseconds to wait=20) -> ()  [unwired: 1 out]
        n191 = Greater Or Equal?(x=w410, y=w374) -> (x >= y?=w407:bool)
        n192 = call-poly <vilib>:"PID.vi"("output range"=w397, "dt (s)"=0.01 ("proportional gain (Kc)"), "PID gains"=w387, "process variable"=w383, "setpoint"=w377) -> ("output"=w384:dbl)  [unwired: 5 in, 1 out]
        n193 = call-poly <vilib>:"WPI_RobotDriveArcadeDrive.vi"("Y axis value"=0.0, "X axis value"=w384, "RobotDriveDevRef"=w406) -> ("RobotDriveDevRef"=w405:T6)  [unwired: 1 in, 7 out]
        n194 = call-poly <vilib>:"NT Write Value.vi"("Numeric"=w384, "Name"="X-Axis" ("refnum name")) -> ()  [unwired: 9 in, 1 out]
      }
      n195 = while {
        tunnel: w363 -> [w412]
        tunnel: [w411] -> _
        stop <- FALSE stop-if-true
        # "stand still"
        n196 = call-poly <vilib>:"WPI_RobotDriveArcadeDrive.vi"("Y axis value"=0.0 ("X axis value"), "X axis value"=0.0, "RobotDriveDevRef"=w412) -> ("RobotDriveDevRef"=w411:T6)  [unwired: 1 in, 7 out]
        n197 = Wait (ms)(milliseconds to wait=20) -> ()  [unwired: 1 out]
      }
    }
    frame "Drive Straight Gyro Set From Dashboard" {
      # "5 Seconds"
      n198 = call <vilib>:"WPI_GyroRefNum Registry Get.vi"("refnum name"="Gyro") -> ("error out"=w418:errorcluster, "GyroDevRef"=w419:T13)  [unwired: 9 in]
      n199 = call <vilib>:"WPI_SolenoidRefNum Registry Get.vi"("refnum name"="Gear Holder") -> ("SolenoidDevRef"=w423:T11)  [unwired: 9 in, 1 out]
      n200 = call <vilib>:"WPI_RobotDriveRefNum Registry Get.vi"("refnum name"="Left and Right Motors") -> ("RobotDriveDevRef"=w427:T6)  [unwired: 1 in, 9 out]
      n201 = call-poly <vilib>:"WPI_SolenoidSet.vi"("Value"=WPI_SolenoidValue."Reverse", "SolenoidDevRef"=w423) -> ("error out"=w425:errorcluster, "SolenoidDevRef"=w424:T11)  [unwired: 8 in]
      n202 = call <vilib>:"WPI_GyroReset.vi"("error in"=w418, "GyroDevRef"=w419) -> ("GyroDevRef"=w417:T13)  [unwired: 8 in, 1 out]
      n203 = call-poly <vilib>:"WPI_SolenoidGet.vi"("error in (no error)"=w425, "SolenoidDevRef"=w424) -> ()  [unwired: 7 in, 3 out]
      n204 = while {
        tunnel: w427 -> [w460]
        tunnel: [w459] -> w421
        tunnel: w417 -> [w429]
        i -> [w463]
        stop <- w461 stop-if-true
        # "P\nI\nD"
        n205 = call <vilib>:"WPI_GyroGetAngle.vi"("GyroDevRef"=w429) -> ("Angle"=w437:dbl, "Calibrated?"=→"Boolean 3":bool)  [unwired: 6 in, 3 out]
        n206 = call-poly <vilib>:"NT Read Value.vi"("Default Value"=4.0, "Name"="T1" ("refnum name")) -> ("Numeric"=w431:dbl)  [unwired: 8 in, 1 out]
        n207 = Increment(x=w463) -> (x+1=w464:i32)
        n208 = Wait (ms)(milliseconds to wait=20) -> ()  [unwired: 1 out]
        n209 = Multiply(x=w431, y=50.0) -> (x*y=w430:dbl)
        n210 = Greater Or Equal?(x=w464, y=w430) -> (x >= y?=w461:bool)
        n211 = call-poly <vilib>:"NT Read Value.vi"("Default Value"=0.8, "Name"="Range Low" ("refnum name")) -> ("Numeric"=w452:dbl)  [unwired: 8 in, 1 out]
        n212 = call-poly <vilib>:"NT Read Value.vi"("Default Value"=0.8, "Name"="Range High" ("refnum name")) -> ("Numeric"=w453:dbl)  [unwired: 8 in, 1 out]
        n213 = call-poly <vilib>:"NT Read Value.vi"("Default Value"=10.0, "Name"="I" ("refnum name")) -> ("Numeric"=w444:dbl)  [unwired: 8 in, 1 out]
        n214 = call-poly <vilib>:"NT Read Value.vi"("Default Value"=0.0, "Name"="D" ("refnum name")) -> ("Numeric"=w443:dbl)  [unwired: 8 in, 1 out]
        n215 = call-poly <vilib>:"NT Read Value.vi"("Default Value"=0.3, "Name"="P" ("refnum name")) -> ("Numeric"=w442:dbl)  [unwired: 8 in, 1 out]
        n216 = Bundle("Numeric"=w442, "Numeric"=w444, "Numeric"=w443) -> (w441:T16)  [unwired: 1 in]
        n217 = Bundle("Numeric"=w453, "Numeric"=w452) -> (w451:cluster{"Numeric":dbl, "Numeric":dbl})  [unwired: 1 in]
        n218 = call-poly <vilib>:"PID.vi"("output range"=w451, "dt (s)"=0.01 ("proportional gain (Kc)"), "PID gains"=w441, "process variable"=w437, "setpoint"=0.0) -> ("output"=w438:dbl)  [unwired: 5 in, 1 out]
        n219 = call-poly <vilib>:"WPI_RobotDriveArcadeDrive.vi"("Y axis value"=0.8, "X axis value"=w438, "RobotDriveDevRef"=w460) -> ("RobotDriveDevRef"=w459:T6)  [unwired: 1 in, 7 out]
        n220 = call-poly <vilib>:"NT Write Value.vi"("Numeric"=w438, "Name"="X-Axis" ("refnum name")) -> ()  [unwired: 9 in, 1 out]
      }
      n221 = while {
        tunnel: w421 -> [w466]
        tunnel: [w465] -> _
        stop <- FALSE stop-if-true
        # "stand still"
        n222 = call-poly <vilib>:"WPI_RobotDriveArcadeDrive.vi"("Y axis value"=0.0 ("X axis value"), "X axis value"=0.0, "RobotDriveDevRef"=w466) -> ("RobotDriveDevRef"=w465:T6)  [unwired: 1 in, 7 out]
        n223 = Wait (ms)(milliseconds to wait=20) -> ()  [unwired: 1 out]
      }
    }
  }
  n224 = Index Array(array=w2, index=2) -> ()  [unwired: 1 out]
  n225 = call-poly <vilib>:"NT Write Value.vi"("Numeric Array"=w2, "Name"="Joystick 0/Axes") -> ()  [unwired: 9 in, 1 out]
